vi "Set Image from Picture.vi"(7 "Button Size":i32, 8 "error in (no error)":errorcluster, 9 "State":T1, 10 "Picture":picture, 11 "Button in":refnum<class "Button.lvclass">) -> (0 "error out":errorcluster, 3 "Button out":refnum<class "Button.lvclass">)   [LabVIEW 2012, in "Button.lvclass"]
uses:
  Button.lvclass
  Type Defs/Button Status.ctl
  Button.lvclass/Button.ctl
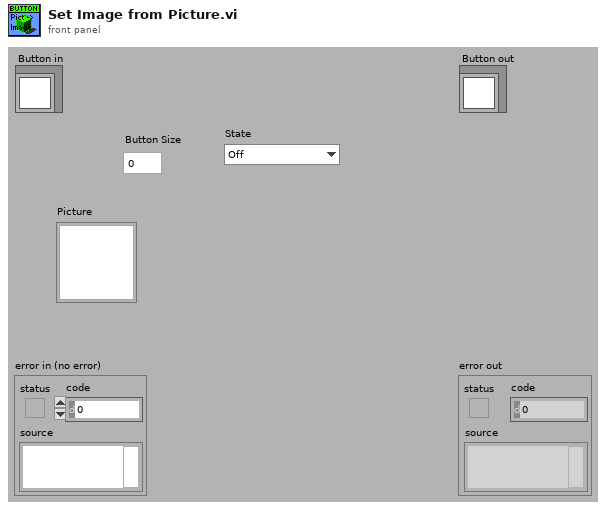
[diagram p1: front panel]
types:
  T1 = typedef "Button.lvclass/Button Status.ctl" = enum16{"Off", "Hover", "On", "Disabled"}
  T2 = typedef "imagedata.ctl" = cluster{"image type":i32, "image depth":i32, "image":u8[], "mask":u8[], "colors":u32[], "Rectangle":cluster{"left":i16, "top":i16, "right":i16, "bottom":i16}}
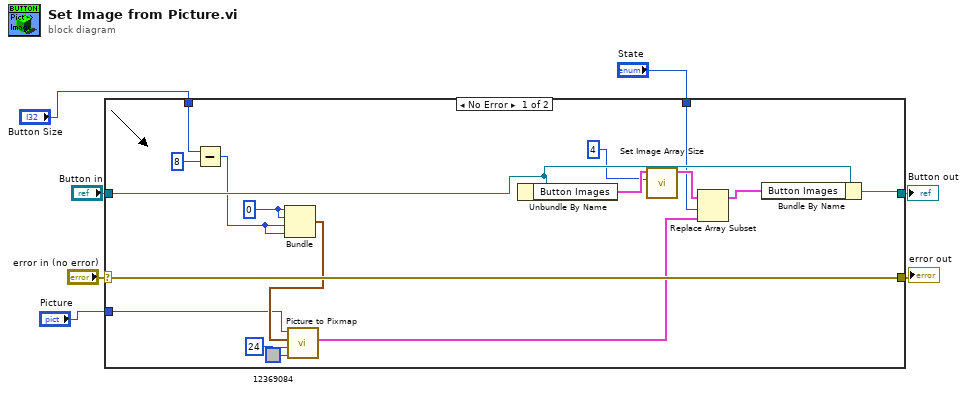
[diagram p0: block diagram]
diagram:
  n1 = case shown="No Error" "error in (no error)" {
    selector: "error in (no error)" -> [w24 w26]
    tunnel: [w24 w26] -> w6
    tunnel: [w14 w25] -> w4
    tunnel: "Button in" -> [w16 w25]
    tunnel: "Picture" -> [w15 _]
    tunnel: "Button Size" -> [w11 _]
    tunnel: "State" -> [w10 _]
    frame No Error {
      w21 = 0
      n2 = Subtract(x=w11, y=8) -> (x-y=w12:i32)
      n3 = Bundle(w21, w21, w12, w12) -> (w20:cluster{i32, i32, i32, i32})  [unwired: 1 out]
      n4 = call <vilib>:"Picture to Pixmap.vi"("Background Color"=u32 12369084, "depth"=24, "rect"=w20, "picture"=w15) -> ("image data"=w18:T2)  [unwired: 7 out]
      n5 = Unbundle By Name(w16) -> ("Button Images"=w9:T2[])
      n6 = call "Set Image Array Size.vi"("Buttons Displayed"=4, "Button Images in"=w9) -> ("Button Images out"=w17:T2[])  [unwired: 9 in]
      n7 = Replace Array Subset(array=w17, new element=w18, index=w10) -> (w19:T2[])
      n8 = Bundle By Name(cluster=w16, "Button Images"=w19) -> (w14:refnum<class "Button.lvclass">)
    }
    frame Error {
    }
  }
  "error out" <- w6
  "Button out" <- w4
